vi "MouseZoomY.vi"(8 "YNum":i32, 9 "Coords":T1, 10 "Delta":i32, 11 "XYGraph输入":refnum<vi>) -> ()   [LabVIEW 2015]
uses:
  <vilib>/Utility/miscctls.llb/LVPoint32TypeDef.ctl
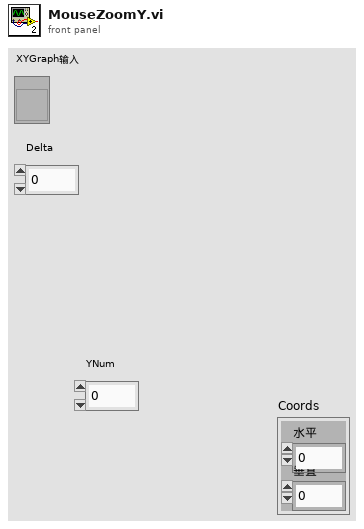
[diagram p1: front panel]
types:
  T1 = typedef "LVPoint32TypeDef.ctl" = cluster{"Horizontal":i32, "Vertical":i32}
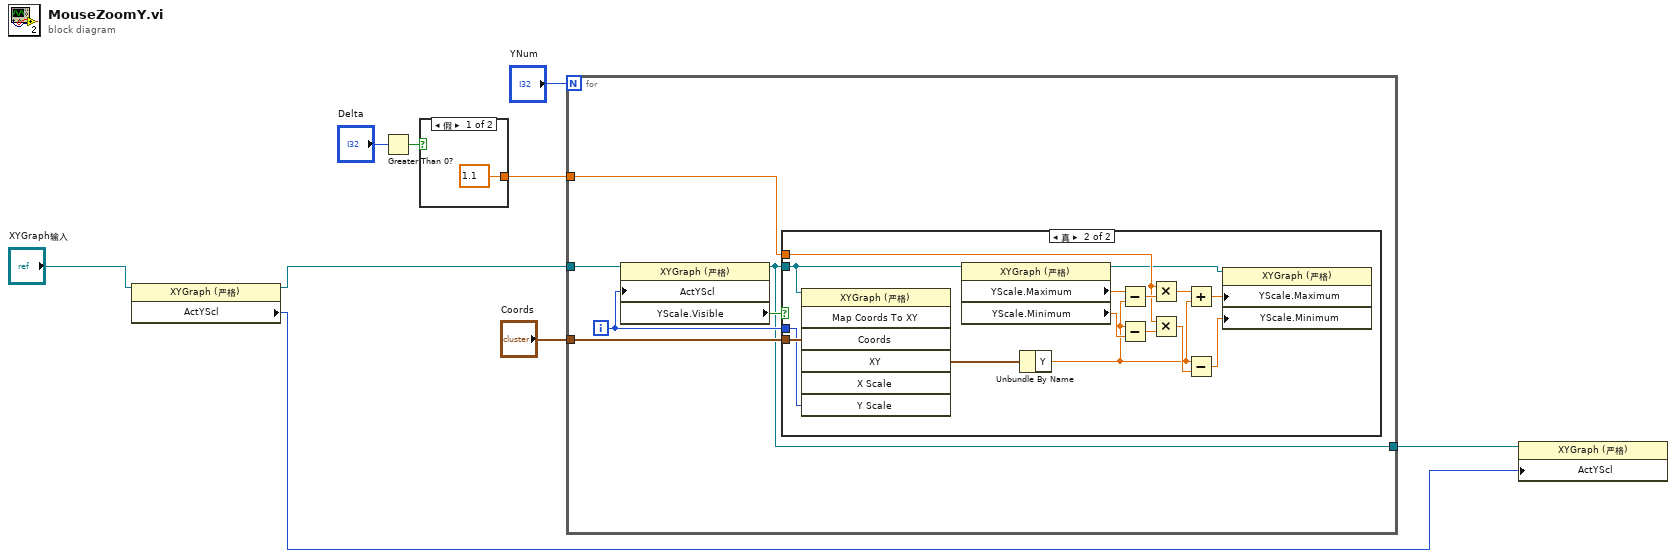
[diagram p0: block diagram]
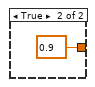
[diagram p3: hidden frame]
diagram:
  n1 = property class="XYGraph (严格)"(reference="XYGraph输入") -> (reference out=w3:refnum<vi>, "ActYScl"=w1:i32)  [unwired: 1 in, 1 out]
  n2 = Greater Than 0?(x="Delta") -> (x > 0?=w9:bool)
  n3 = case shown="假" w9 {
    tunnel: [1.1 0.9] -> w7
    frame False {
    }
    frame True {
    }
  }
  n4 = for {
    N: "YNum" -> [_]
    tunnel: w3 -> [w15]
    tunnel: w7 -> [w17]
    tunnel: "Coords" -> [w14]
    tunnel: [w12] -> w2
    i -> [w13]
    n5 = property class="XYGraph (严格)"(reference=w15, "ActYScl"=w13) -> (reference out=w12:refnum<vi>, "YScale.Visible"=w16:bool)  [unwired: 1 in, 1 out]
    n6 = case shown="真" w16 {
      tunnel: w12 -> [_ w22]
      tunnel: w17 -> [_ w28]
      tunnel: w14 -> [_ w21]
      tunnel: w13 -> [_ w20]
      frame False {
      }
      frame True {
        n7 = invoke class="XYGraph (严格)" method="Map Coords To XY"(reference=w22, "Coords"=w21, "Y Scale"=w20) -> ("XY"=w19:cluster{"X":dbl, "Y":dbl})  [unwired: 4 in, 6 out]
        n8 = property class="XYGraph (严格)"(reference=w22) -> (reference out=w25:refnum<vi>, "YScale.Maximum"=w24:dbl, "YScale.Minimum"=w30:dbl)  [unwired: 1 in, 1 out]
        n9 = Unbundle By Name(w19) -> ("Y"=w18:dbl)
        n10 = Subtract(x=w24, y=w18) -> (x-y=w32:dbl)
        n11 = Subtract(x=w18, y=w30) -> (x-y=w29:dbl)
        n12 = Multiply(x=w28, y=w32) -> (x*y=w31:dbl)
        n13 = Multiply(x=w28, y=w29) -> (x*y=w27:dbl)
        n14 = Add(x=w31, y=w18) -> (x+y=w23:dbl)
        n15 = Subtract(x=w18, y=w27) -> (x-y=w26:dbl)
        n16 = property class="XYGraph (严格)"(reference=w25, "YScale.Maximum"=w23, "YScale.Minimum"=w26) -> ()  [unwired: 1 in, 2 out]
      }
    }
  }
  n17 = property class="XYGraph (严格)"(reference=w2, "ActYScl"=w1) -> ()  [unwired: 1 in, 2 out]
